vi "Velocity.vi"(8 "Error In":errorcluster, 10 "Number of pulses":i32, 11 "LINX Resource IN":T1) -> (0 "Error Out":errorcluster, 1 "RPM":dbl, 2 "Velocity (Degrees/Seconds)":dbl, 3 "LINX Resource OUT":T1, 4 "dt":dbl, 5 "Position (Degrees)":dbl)   [LabVIEW 2016]
uses:
  <vilib>/MakerHub/LINX/Private/Type Defs/LINX Ref.ctl
  <vilib>/MakerHub/LINX/Private/Type Defs/Platform.ctl
  <vilib>/MakerHub/LINX/Private/Type Defs/Interface.ctl
  <vilib>/MakerHub/LINX/Private/Device/Type Defs/LINX Device Config.ctl
  <vilib>/MakerHub/LINX/Private/Device/Type Defs/TCP Config.ctl
  <vilib>/MakerHub/LINX/Private/Device/Type Defs/Channels.ctl
  <vilib>/MakerHub/LINX/LMH-LINX.lvlib
  <vilib>/MakerHub/LINX/Private/Device/Device.lvlib
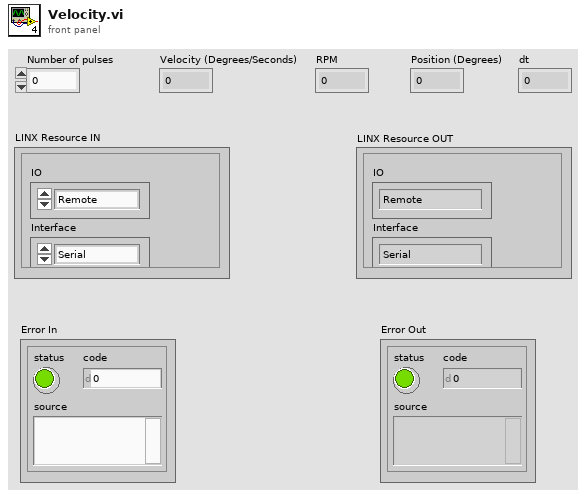
[diagram p1: front panel]
types:
  T1 = typedef "LMH-LINX.lvlib/LINX Ref.ctl" = cluster{"IO":T2, "Interface":T3, "LINX Device Config":T4}
  T2 = typedef "LMH-LINX.lvlib/Platform.ctl" = enum16{"Remote", "Local"}
  T3 = typedef "LMH-LINX.lvlib/Interface.ctl" = enum16{"Serial", "TCP"}
  T4 = typedef "LMH-LINX.lvlib/Device.lvlib/LINX Device Config.ctl" = cluster{"Interface":T3, "COM Port":refnum<visa-resource-name>, "TCP Configuration":T5, "Device Family":u8, "Device ID":u8, "Device Name":string, "TCP Ref":refnum<k5>, "Channels":T6}
  T5 = typedef "LMH-LINX.lvlib/Device.lvlib/TCP Config.ctl" = cluster{"IP Address":string, "Port":u16}
  T6 = typedef "LMH-LINX.lvlib/Channels.ctl" = cluster{"DI":u8[], "DO":u8[], "AI":u8[], "AO":u8[], "PWM":u8[], "QE":u8[], "UART":u8[], "I2C 2":u8[], "SPI":u8[], "CAN":u8[], "Servo":u8[], "AI Ref (V)":dbl, "AI Resolution (Bits)":u8, "AO Ref (V)":dbl, "AO Resolution (Bits)":u8}
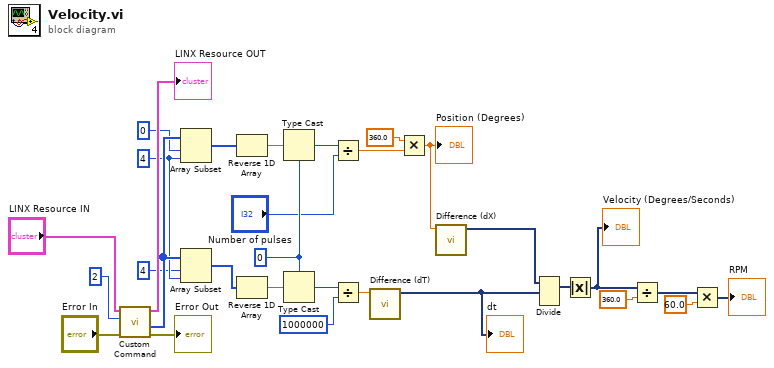
[diagram p0: block diagram]
diagram:
  w19 = 0
  w24 = 4
  n1 = call <vilib>:"Custom Command.vi"("Error In"="Error In", "Custom Command Number"=u16 2, "LINX Resource"="LINX Resource IN") -> ("Error Out"=→"Error Out":errorcluster, "Response"=w25:u8[], "LINX Resource"=→"LINX Resource OUT":T1)  [unwired: 5 in, 1 out]
  n2 = Array Subset(array=w25, index=0, length=w24) -> (w21:u8[])
  n3 = Array Subset(array=w25, index=4, length=w24) -> (w20:u8[])
  n4 = Reverse 1D Array(array=w21) -> (reversed array=w17:u8[])
  n5 = Reverse 1D Array(array=w20) -> (reversed array=w18:u8[])
  n6 = Type Cast(type=w19, x=w17) -> (*(type *) &x=w15:i32)
  n7 = Type Cast(type=w19, x=w18) -> (*(type *) &x=w11:i32)
  n8 = Divide(x=w15, y="Number of pulses") -> (x/y=w13:dbl)
  n9 = Divide(x=w11, y=1000000) -> (x/y=w8:dbl)
  n10 = call "Difference (dT)"("Signals"=w8) -> ("Result"=w1:dynamicdata)  [unwired: 5 in, 1 out]
  "dt" <- w1
  n11 = Multiply(x=360.0, y=w13) -> (x*y=w9:dbl)
  "Position (Degrees)" <- w9
  n12 = call "Difference (dX)"("Signals"=w9) -> ("Result"=w16:dynamicdata)  [unwired: 5 in, 1 out]
  n13 = Divide(1:w1, 2:w16) -> (0:w3:dynamicdata)  [unwired: 1 in, 1 out]
  n14 = Absolute Value(x=w3) -> (abs(x)=w2:dynamicdata)
  "Velocity (Degrees/Seconds)" <- w2
  n15 = Divide(x=w2, y=360.0) -> (x/y=w5:dynamicdata)
  n16 = Multiply(x=w5, y=60.0) -> (x*y=→"RPM":dynamicdata)
